vi "Analysis.vi"(8 "error in (no error)":errorcluster, 11 "Hot And Cold Source Unit Model in":refnum<class "Hot And Cold Source Unit Model.lvclass">) -> (0 "error out":errorcluster, 3 "Hot And Cold Source Unit Model out":refnum<class "Hot And Cold Source Unit Model.lvclass">)   [LabVIEW 2013, in "Hot And Cold Source Unit Model.lvlib" / "Hot And Cold Source Unit Model.lvclass"]
uses:
  Hot And Cold Source Unit Model.lvclass
  Hot And Cold Source Unit Model.lvclass/Hot And Cold Source Unit Model.ctl
  Common/Parameter/Abstract Sensor Parameter/Abstract Sensor Parameter.lvclass
  Common/Parameter/Abstract Sensor Parameter/Abstract Sensor Parameter.lvclass/Abstract Sensor Parameter.ctl
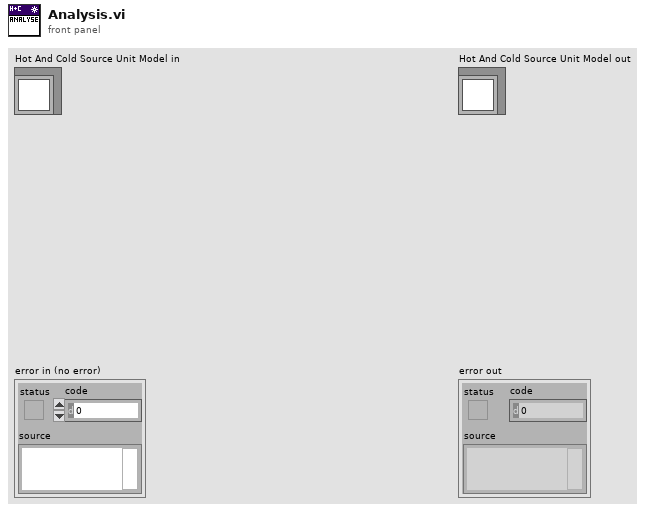
[diagram p1: front panel]
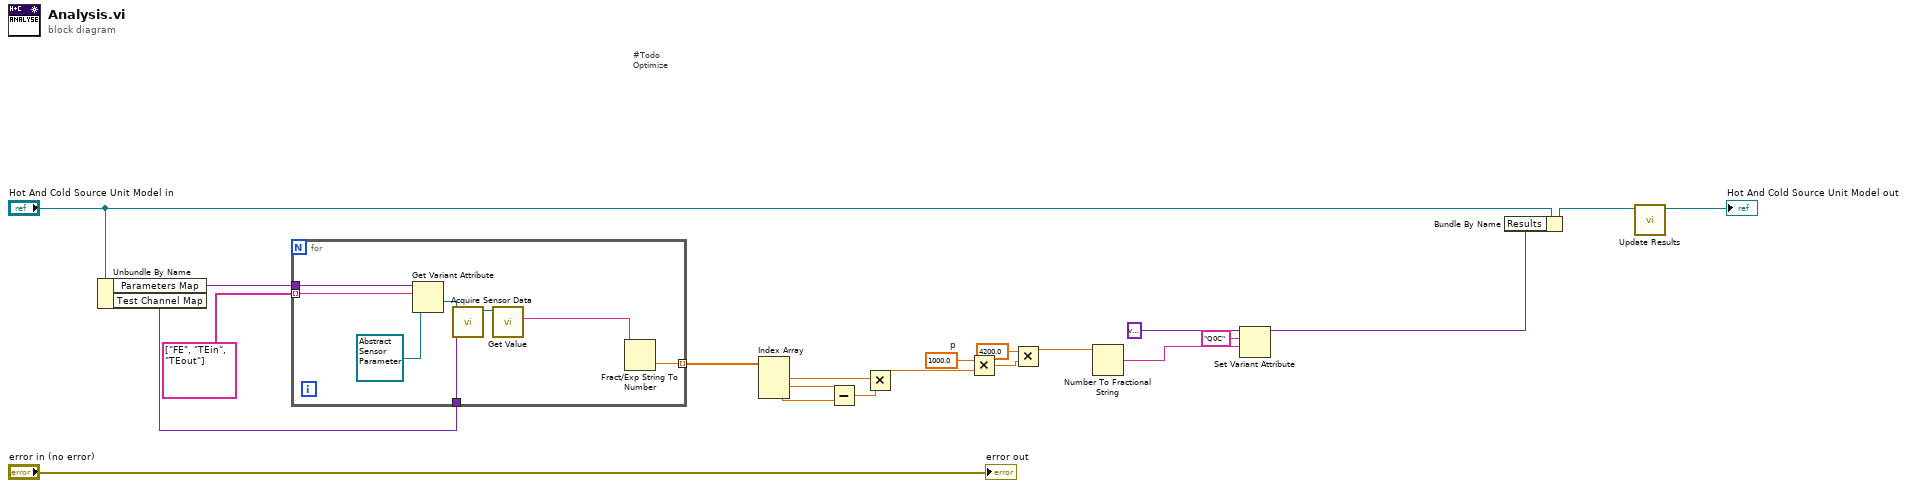
[diagram p0: block diagram]
diagram:
  w10 = 1000.0  # p
  # "#Todo\nOptimize"
  n1 = Unbundle By Name("Hot And Cold Source Unit Model in") -> ("Parameters Map"=w21:variant, "Test Channel Map"=w18:variant)
  n2 = for {
    tunnel: w21 -> [w29]
    tunnel: w18 -> [w25]
    tunnel: [w23] -> w16 mode=indexing
    tunnel: string[] ["FE", "TEin", "TEout"] -> [w22] mode=indexing
    n3 = Get Variant Attribute(Variant=w29, name=w22, default value (empty Variant)=refnum<class "Abstract Sensor Parameter.lvclass"> refnum ("Parameter.lvlib:Abstract Sensor Parameter.lvclass")) -> (value=w24:refnum<class "Abstract Sensor Parameter.lvclass">)  [unwired: 1 in, 3 out]
    n4 = call-dynamic "Acquire Sensor Data.vi"("Test Channel Map"=w25, "Abstract Sensor Parameter in"=w24) -> ("Abstract Sensor Parameter out"=w27:refnum<class "Abstract Sensor Parameter.lvclass">)  [unwired: 8 in, 1 out]
    n5 = call "Get Value.vi"("Parameter in"=w27) -> ("Value"=w26:string)  [unwired: 8 in, 2 out]
    n6 = Fract/Exp String To Number(string=w26) -> (number=w23:dbl)  [unwired: 3 in, 1 out]
  }
  n7 = Index Array(array=w16) -> (element #1=w13:dbl, element #2=w15:dbl, element #3=w14:dbl)  [unwired: 3 in]
  n8 = Subtract(x=w15, y=w14) -> (x-y=w12:dbl)
  n9 = Multiply(x=w13, y=w12) -> (x*y=w11:dbl)
  n10 = Multiply(x=w10, y=w11) -> (x*y=w9:dbl)
  n11 = Multiply(x=4200.0, y=w9) -> (x*y=w7:dbl)
  n12 = Number To Fractional String(number=w7) -> (F-format string=w6:string)  [unwired: 3 in]
  n13 = Set Variant Attribute(Variant=variant, name="Q0C", value=w6) -> (Variant out=w3:variant)  [unwired: 1 in, 2 out]
  n14 = Bundle By Name(cluster="Hot And Cold Source Unit Model in", "Results"=w3) -> (w4:refnum<class "Hot And Cold Source Unit Model.lvclass">)
  n15 = call "Update Results.vi"("Hot And Cold Source Unit Model in"=w4) -> ("Hot And Cold Source Unit Model out"=→"Hot And Cold Source Unit Model out":refnum<class "Hot And Cold Source Unit Model.lvclass">)  [unwired: 9 in, 1 out]
  "error out" <- "error in (no error)"
